vi "RLS_Phase_Estimator.vi"(2 "Frequency Estimator Settings":T1, 3 "u":sgl, 4 "theta":sgl, 5 "wcs":sgl) -> (0 "uphq":sgl, 1 "uphd":sgl)   [LabVIEW 2013]
uses:
  FreqEstimator.ctl
  <vilib>/rvi/FXPMathLib/FxpSinAndCos/subVIs/nifxpmath_SinAndCos_SimConfig.ctl
  <vilib>/rvi/FXPMathLib/FxpSinAndCos/simVIs/DllFxpSinAndCosTemp_sub.vi
  <vilib>/rvi/FXPMathLib/FxpSinAndCos/XNode/nifxpmath_SinAndCos.xnode
panel:
  out "innov":sgl
  # "This VI is configured as Non-reentrant. \nOnly ONE copy of the Vi actually exists on the FPGA hardware."
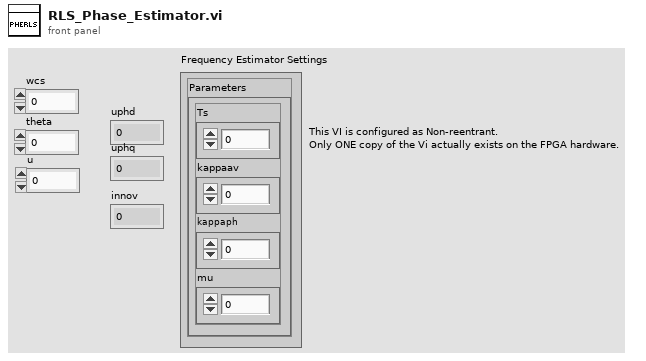
[diagram p1: front panel]
types:
  T1 = typedef "FreqEstimator.ctl" = cluster{"Parameters":cluster{"Ts":sgl, "kappaav":sgl, "kappaph":sgl, "mu":sgl}}
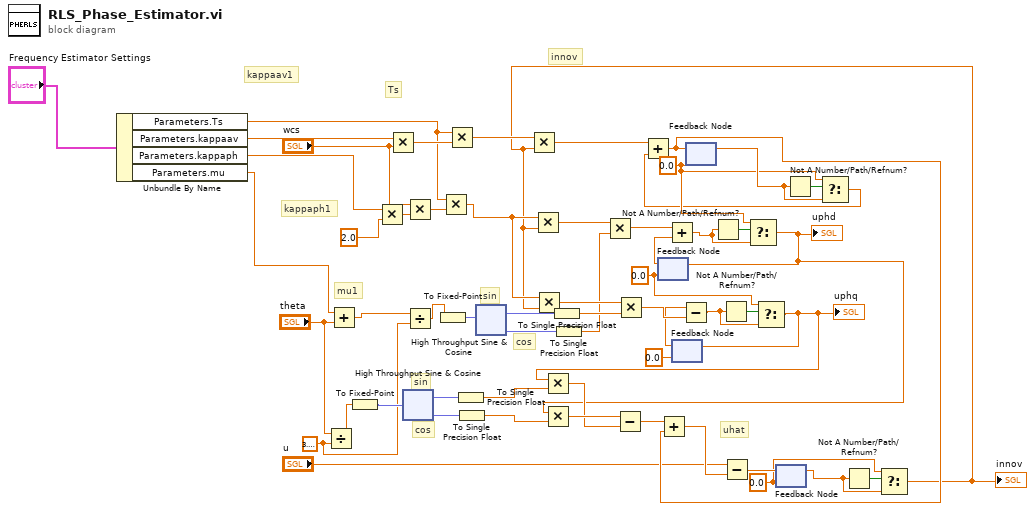
[diagram p0: block diagram]
diagram:
  w13 = sgl 0.0
  w9 = sgl 0.0
  w2 = sgl 0.0
  w19 = sgl 3.1415927
  # "cos"
  # "sin"
  # "uhat"
  # "sin"
  # "cos"
  # "mu1"
  # "kappaph1"
  # "innov"
  # "kappaav1"
  # "Ts"
  n1 = Unbundle By Name("Frequency Estimator Settings") -> ("Parameters.Ts"=w22:sgl, "Parameters.kappaav"=w25:sgl, "Parameters.kappaph"=w24:sgl, "Parameters.mu"=w23:sgl)
  n2 = Divide(x="theta", y=w19) -> (x/y=w16:sgl)
  n3 = Add(x=w23, y="theta") -> (x+y=w20:sgl)
  n4 = To Fixed-Point(number=w16) -> (fixed-point=w36:fxp<+/-,44,24>)  [unwired: 1 in]
  n5 = Multiply(x=w24, y=sgl 2.0) -> (x*y=w53:sgl)
  n6 = Multiply(x=w25, y="wcs") -> (x*y=w57:sgl)
  n7 = xnode "High Throughput Sine & Cosine"("x (pi)"=w36) -> ("sin(x)"=w35:fxp<+/-,44,2>, "cos(x)"=w34:fxp<+/-,44,2>)
  n8 = Multiply(x="wcs", y=w53) -> (x*y=w51:sgl)
  n9 = Divide(x=w20, y=w19) -> (x/y=w17:sgl)
  n10 = To Fixed-Point(number=w17) -> (fixed-point=w31:fxp<+/-,44,24>)  [unwired: 1 in]
  n11 = Multiply(x=w22, y=w51) -> (x*y=w47:sgl)
  n12 = Multiply(x=w22, y=w57) -> (x*y=w56:sgl)
  n13 = To Single Precision Float(number=w35) -> (single precision float=w33:sgl)
  n14 = To Single Precision Float(number=w34) -> (single precision float=w32:sgl)
  n15 = xnode "High Throughput Sine & Cosine"("x (pi)"=w31) -> ("sin(x)"=w30:fxp<+/-,44,2>, "cos(x)"=w28:fxp<+/-,44,2>)
  n16 = To Single Precision Float(number=w30) -> (single precision float=w29:sgl)
  n17 = To Single Precision Float(number=w28) -> (single precision float=w27:sgl)
  n18 = feedback #1(w9) -> (w48:sgl)
  n19 = feedback #2(sgl 0.0) -> (w44:sgl)
  n20 = feedback #3(w2) -> (w3:sgl)
  n21 = feedback #4(w13) -> (w14:sgl)
  n22 = Not A Number/Path/Refnum?(number/path/refnum=w3) -> (NaN/Path/Refnum?=w4:bool)
  n23 = Select(t=w2, s=w4, f=w3) -> (s? t:f=w1:sgl)
  n24 = Not A Number/Path/Refnum?(number/path/refnum=w14) -> (NaN/Path/Refnum?=w15:bool)
  n25 = Select(t=w13, s=w15, f=w14) -> (s? t:f=w12:sgl)
  "innov" <- w12
  n26 = Multiply(x=w56, y=w12) -> (x*y=w55:sgl)
  n27 = Multiply(x=w47, y=w12) -> (x*y=w50:sgl)
  n28 = Multiply(x=w47, y=w12) -> (x*y=w46:sgl)
  n29 = Multiply(x=w50, y=w27) -> (x*y=w49:sgl)
  n30 = Multiply(x=w46, y=w29) -> (x*y=w45:sgl)
  n31 = Add(x=w55, y=w1) -> (x+y=w40:sgl)
  n32 = Add(x=w49, y=w48) -> (x+y=w6:sgl)
  n33 = Subtract(x=w44, y=w45) -> (x-y=w10:sgl)
  n34 = feedback-in #3(w40) -> ()
  n35 = Not A Number/Path/Refnum?(number/path/refnum=w6) -> (NaN/Path/Refnum?=w7:bool)
  n36 = Not A Number/Path/Refnum?(number/path/refnum=w10) -> (NaN/Path/Refnum?=w11:bool)
  n37 = Select(t=w2, s=w7, f=w6) -> (s? t:f=w5:sgl)
  "uphd" <- w5
  n38 = Multiply(x=w5, y=w32) -> (x*y=w43:sgl)
  n39 = feedback-in #1(w5) -> ()
  n40 = Select(t=w9, s=w11, f=w10) -> (s? t:f=w8:sgl)
  "uphq" <- w8
  n41 = Multiply(x=w8, y=w33) -> (x*y=w42:sgl)
  n42 = Subtract(x=w43, y=w42) -> (x-y=w41:sgl)
  n43 = Add(x=w41, y=w40) -> (x+y=w39:sgl)
  n44 = feedback-in #2(w8) -> ()
  n45 = Subtract(x="u", y=w39) -> (x-y=w37:sgl)
  n46 = feedback-in #4(w37) -> ()
